vi "subAxopatch_ApplySealTestWave.vi"(5 "samples":i32=40000, 6 "Patch  Ex. Commnd AO Line":tag="Dev1/ao0" caption="Patch Ex. Command AO Line", 7 "Sampling rate (Hz)":dbl=20000.0 format="%0.2f", 8 "error in":errorcluster, 9 "Dev1 Trigger source":tag="/Dev1/PFI0", 10 "Patch AI lines 1":T1={"Scaled output line"="Dev1/ai8", "10 V_m line"="Dev1/ai0"}, 11 "Patch seal test waveform":waveform(dbl)(graph)={"t0"=timestamp(0 s since 1904-01-01), "dt"=5e-05, "Y"=array[40000 elements]}) -> (0 "error out":errorcluster={"status"=TRUE, "code"=-200284, "source"="subAxopatch_ApplySealTestWave.vi<append>\n<B>Property: </B>RelativeTo\n<B>Requested Value: </B>Current Read Position\n\n<B>Property: </B>Offset\n<B>Requested Value: </B>0\n\n<B>Task Name: </B>_unnamedTask<3>"}, 2 "Scaled output":cluster{"xo":i32, dbl, "data":dbl[][]}(graph)={"xo"=0, 5e-05, "data"=[]}, 3 "AI data":dbl[][](graph))   [LabVIEW 2015]
uses:
  <vilib>/DAQmx/write.llb/DAQmx Write (Analog Wfm 1Chan NSamp).vi
  <vilib>/DAQmx/read.llb/DAQmx Read (Analog 2D DBL NChan NSamp).vi
  <vilib>/DAQmx/create/channels.llb/DAQmx Create Channel (AO-Voltage-Basic).vi
  <vilib>/DAQmx/configure/timing.llb/DAQmx Timing (Sample Clock).vi
  <vilib>/DAQmx/configure/trigger.llb/DAQmx Start Trigger (Digital Edge).vi
  <vilib>/DAQmx/miscellaneous.llb/DAQmx Fill In Error Info.vi
  <vilib>/DAQmx/create/channels.llb/DAQmx Create Channel (AI-Voltage-Basic).vi
panel:
  in  "Digital trigger line":tag[](array[tag])=["Dev1/port0/line1"]
  in  "AI config":T2={"V_max"=10.0, "V_min"=-10.0, "terminal config"=10083} {"terminal config" items=["Default"=-1, "RSE"=10083, "Differential"=10106, "Pseudodifferential"=12529]}
  in  "AO config":T2={"V_max"=5.0, "V_min"=-5.0, "terminal config"=10083} {"terminal config" items=["Default"=-1, "RSE"=10083, "Differential"=10106, "Pseudodifferential"=12529]}
  # "DEV1/port0/LINE1\nUse Dev1 to trigger PFI0\nNo terminal, use the default value"
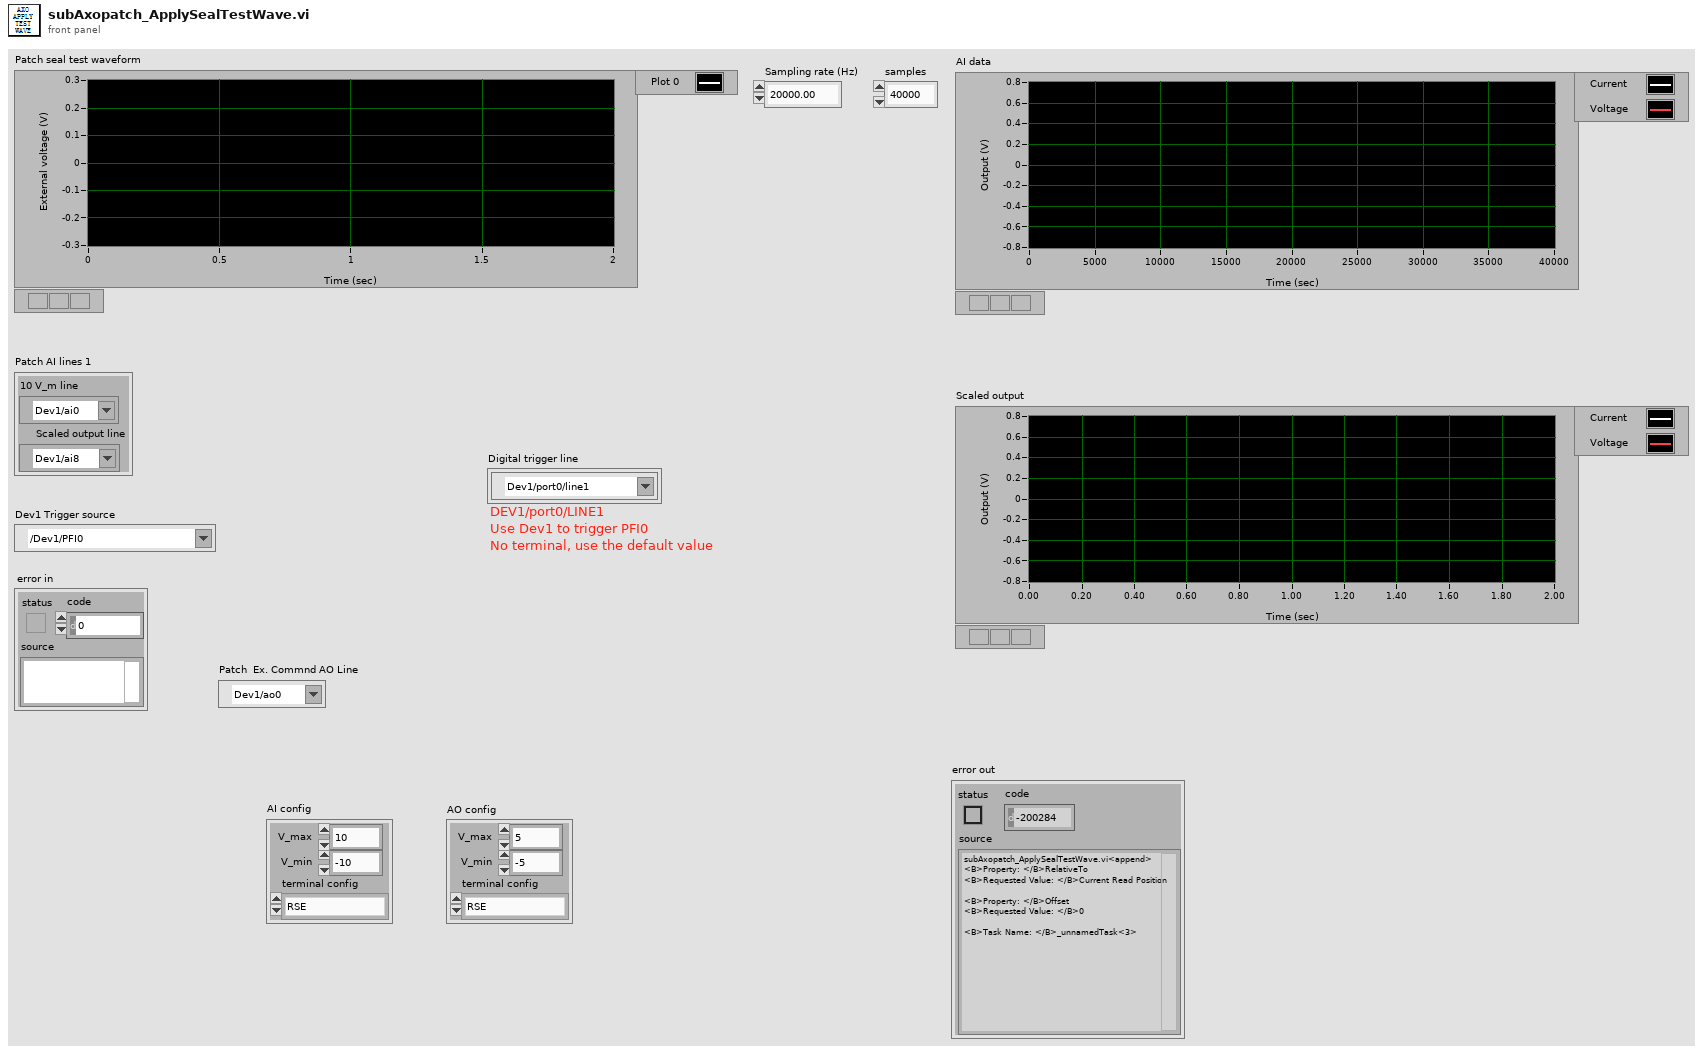
[diagram p1: front panel]
types:
  T1 = cluster{"Scaled output line":tag, "10 V_m line":tag}
  T2 = cluster{"V_max":dbl, "V_min":dbl, "terminal config":i32}
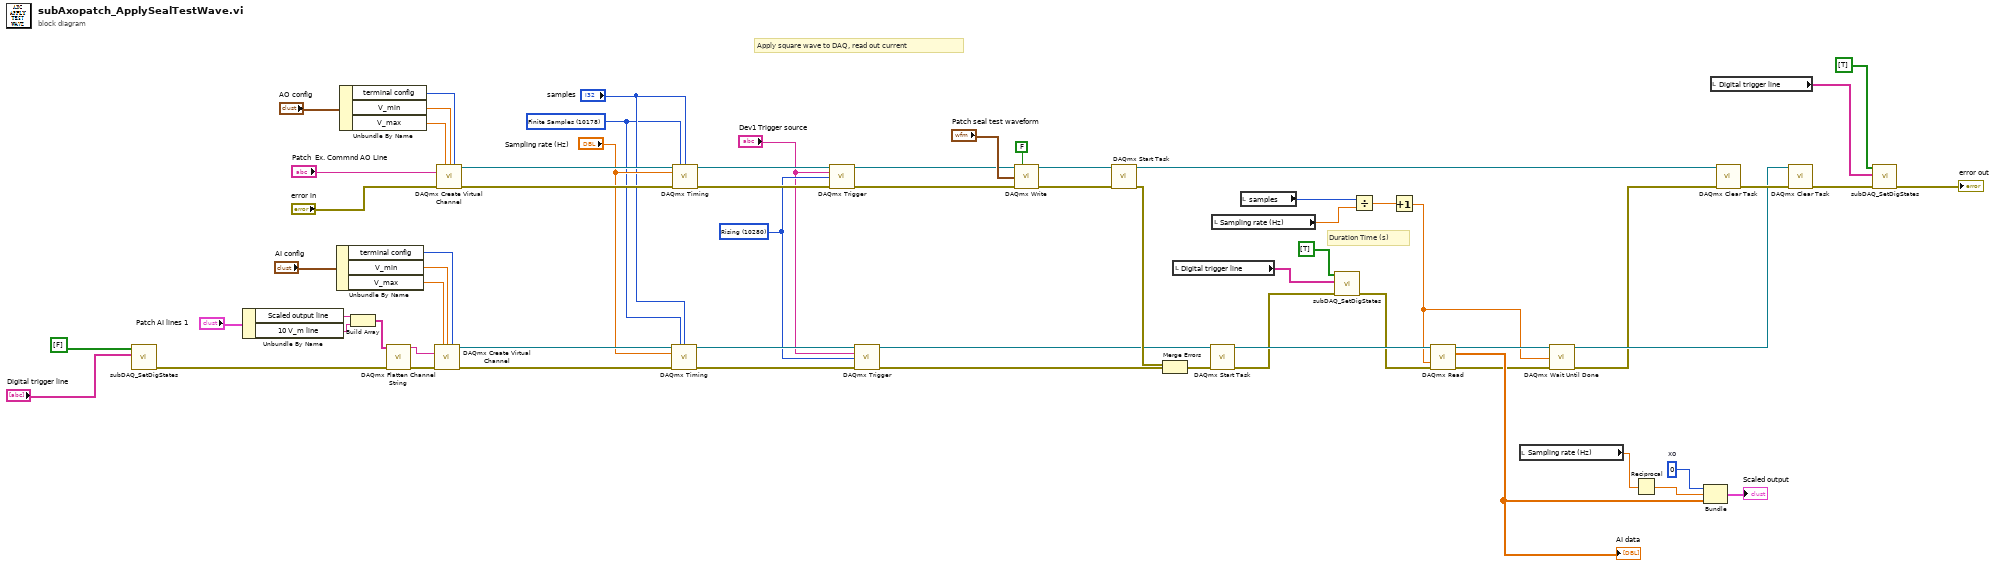
[diagram p0: block diagram]
diagram:
  w24 = 10280 items=["Rising"=10280, "Falling"=10171] ("edge")
  w60 = 0  # xo
  w38 = 10178 items=["Finite Samples"=10178, "Continuous Samples"=10123, "Hardware Timed Single Point"=12522] ("sample mode")
  # "Duration Time (s)"
  # "Apply square wave to DAQ, read out current"
  n1 = call "subDAQ_SetDigStates.vi"("Digital line array"="Digital trigger line", "Digital States (Value) array"=bool[] [FALSE] ("Digital state array")) -> ("Error out"=w15:errorcluster)  [unwired: 9 in]
  n2 = Unbundle By Name("Patch AI lines 1") -> ("Scaled output line"=w22:tag, "10 V_m line"=w21:tag)
  n3 = Unbundle By Name("AI config") -> ("terminal config"=w49:i32, "V_min"=w48:dbl, "V_max"=w47:dbl)
  n4 = Unbundle By Name("AO config") -> ("terminal config"=w52:i32, "V_min"=w51:dbl, "V_max"=w50:dbl)
  n5 = Build Array(w22, w21) -> (w20:tag[])
  n6 = call <vilib>:"DAQmx Flatten Channel String.vi"("names in"=w20, "error in"=w15) -> ("names out"=w19:string, "error out"=w18:errorcluster)  [unwired: 12 in]
  n7 = call-poly <vilib>:"DAQmx Create Virtual Channel.vi"("maximum value"=w47, "minimum value"=w48, "input terminal configuration"=w49, "physical channels"=w19, "error in"=w18) -> ("task out"=w63:refnum<k21>, "error out"=w62:errorcluster)  [unwired: 9 in]
  n8 = call-poly <vilib>:"DAQmx Create Virtual Channel.vi"("maximum value"=w50, "minimum value"=w51, "output terminal configuration"=w52, "physical channels"="Patch  Ex. Commnd AO Line", "error in"="error in") -> ("task out"=w64:refnum<k21>, "error out"=w61:errorcluster)  [unwired: 9 in]
  n9 = call-poly <vilib>:"DAQmx Timing.vi"("task/channels in"=w63, "sample mode"=w38, "samples per channel"="samples", "rate"="Sampling rate (Hz)", "error in"=w62) -> ("task out"=w28:refnum<k21>, "error out"=w27:errorcluster)  [unwired: 9 in]
  n10 = call-poly <vilib>:"DAQmx Timing.vi"("task/channels in"=w64, "sample mode"=w38, "samples per channel"="samples", "rate"="Sampling rate (Hz)", "error in"=w61) -> ("task out"=w32:refnum<k21>, "error out"=w30:errorcluster)  [unwired: 9 in]
  n11 = call-poly <vilib>:"DAQmx Trigger.vi"("task/channels in"=w32, "source"="Dev1 Trigger source", "edge"=w24, "error in"=w30) -> ("task out"=w31:refnum<k21>, "error out"=w29:errorcluster)  [unwired: 10 in]
  n12 = call-poly <vilib>:"DAQmx Trigger.vi"("task/channels in"=w28, "source"="Dev1 Trigger source", "edge"=w24, "error in"=w27) -> ("task out"=w26:refnum<k21>, "error out"=w25:errorcluster)  [unwired: 10 in]
  n13 = call-poly <vilib>:"DAQmx Write.vi"("task/channels in"=w31, "auto start"=FALSE, "data"="Patch seal test waveform", "error in"=w29) -> ("task out"=w36:refnum<k21>, "error out"=w37:errorcluster)  [unwired: 10 out]
  n14 = call <vilib>:"DAQmx Start Task.vi"("task/channels in"=w36, "error in"=w37) -> ("task out"=w33:refnum<k21>, "error out"=w35:errorcluster)  [unwired: 12 in]
  n15 = Merge Errors(w35, w25) -> (w34:errorcluster)
  n16 = local read "Digital trigger line"() -> (w14:tag[])
  n17 = call <vilib>:"DAQmx Start Task.vi"("task/channels in"=w26, "error in"=w34) -> ("task out"=w65:refnum<k21>, "error out"=w7:errorcluster)  [unwired: 12 in]
  n18 = local read "Sampling rate (Hz)"() -> (w3:dbl)
  n19 = local read "samples"() -> (w4:i32)
  n20 = call "subDAQ_SetDigStates.vi"("Error in (no error)"=w7, "Digital line array"=w14, "Digital States (Value) array"=bool[] [TRUE] ("Digital state array")) -> ("Error out"=w6:errorcluster)  [unwired: 8 in]
  n21 = Divide(x=w4, y=w3) -> (x/y=w2:dbl)
  n22 = Increment(x=w2) -> (x+1=w1:dbl)
  n23 = call-poly <vilib>:"DAQmx Read.vi"("task/channels in"=w65, "timeout"=w1, "error in"=w6) -> ("task out"=w41:refnum<k21>, "data"=w57:dbl[][], "error out"=w8:errorcluster)  [unwired: 10 in]
  "AI data" <- w57
  n24 = local read "Sampling rate (Hz)"() -> (w56:dbl)
  n25 = call <vilib>:"DAQmx Wait Until Done.vi"("task/channels in"=w41, "timeout (sec)"=w1, "error in"=w8) -> ("task out"=w40:refnum<k21>, "error out"=w39:errorcluster)  [unwired: 11 in]
  n26 = Reciprocal(x=w56) -> (1/x=w59:dbl)
  n27 = Bundle("xo"=w60, w59, "data"=w57) -> (→"Scaled output":cluster{"xo":i32, dbl, "data":dbl[][]})  [unwired: 1 in]
  n28 = local read "Digital trigger line"() -> (w11:tag[])
  n29 = call <vilib>:"DAQmx Clear Task.vi"("task in"=w33, "error in"=w39) -> ("error out"=w45:errorcluster)  [unwired: 13 in]
  n30 = call <vilib>:"DAQmx Clear Task.vi"("task in"=w40, "error in"=w45) -> ("error out"=w10:errorcluster)  [unwired: 13 in]
  n31 = call "subDAQ_SetDigStates.vi"("Error in (no error)"=w10, "Digital line array"=w11, "Digital States (Value) array"=bool[] [TRUE] ("Digital state array")) -> ("Error out"=→"error out":errorcluster)  [unwired: 8 in]
